vi "Xml_Fill_Default_Experiments.vi"(6 "error in (no error)":errorcluster, 9 "Resources Path":path=path "D:/PIRENEA/TECHNICAL/RESOURCES") -> (0 "error out":errorcluster caption="sortie d'erreur", 3 "EXPERIMENT Inputs":T1={"Setup"="", "Date"="", "User Name"="", "Comment"="", "Experiment Procedures"=[], "Chemical Source"="", "Sample Components"=[], "Species"=[], "Laser 1"={"Used"=TRUE, "Name"="Spectroscopy", "Wavelength"=1000.0, "Energy"=25.0}, "Laser 2"={"Used"=TRUE, "Name"="Spectroscopy", "Wavelength"=1000.0, "Energy"=25.0}, "Laser 3"={"Used"=TRUE, "Name"="Spectroscopy", "Wavelength"=1000.0, "Energy"=25.0}, "Laser 4"={"Used"=TRUE, "Name"="Spectroscopy", "Wavelength"=1000.0, "Energy"=25.0}, "Laser 5"={"Used"=TRUE, "Name"="Spectroscopy", "Wavelength"=1000.0, "Energy"=25.0}, "Lamp 1"={"Used"=TRUE, "Name"="Yag", "Wavelength"=1000.0, "Attenuation"=25.0}, "Lamp 2"={"Used"=TRUE, "Name"="Yag", "Wavelength"=1000.0, "Attenuation"=25.0}, "Gas 1"={"Used"=TRUE, "Name"="Yag", "Pressure"=1000.0}, "Gas 2"={"Used"=TRUE, "Name"="Yag", "Pressure"=1000.0}, "Gas 3"={"Used"=TRUE, "Name"="Yag", "Pressure"=1000.0}, "Gas 4"={"Used"=TRUE, "Name"="Spectroscopy", "Pressure"=1000.0}, "Gas 5"={"Used"=TRUE, "Name"="Spectroscopy", "Pressure"=1000.0}})   [LabVIEW 2018]
doc: "This example demonstrates how to convert a LabVIEW data structure into an XML string using the GXML reference library."
uses:
  controls/EXPERIMENT_Inputs.ctl
  controls/LASER_Inputs.ctl
  controls/LAMP_Inputs.ctl
  controls/GAS_Inputs.ctl
  <vilib>/Utility/config.llb/Read Key (String).vi
  <vilib>/Utility/config.llb/NI_LVConfig.lvlib
panel:
  in  "Chemical Source":string(combo)
  in  "Setup":string
  in  "Species":i32[](listbox)
  in  "Sample Components":i32[](listbox)
  in  "Procedures":i32[](listbox)
  in  "Users":string(combo)
  # "Lasers"
  # "nm"
  # "mJ"
  # "Lamps"
  # "nm"
  # "dB"
  # "Gas"
  # "bar"
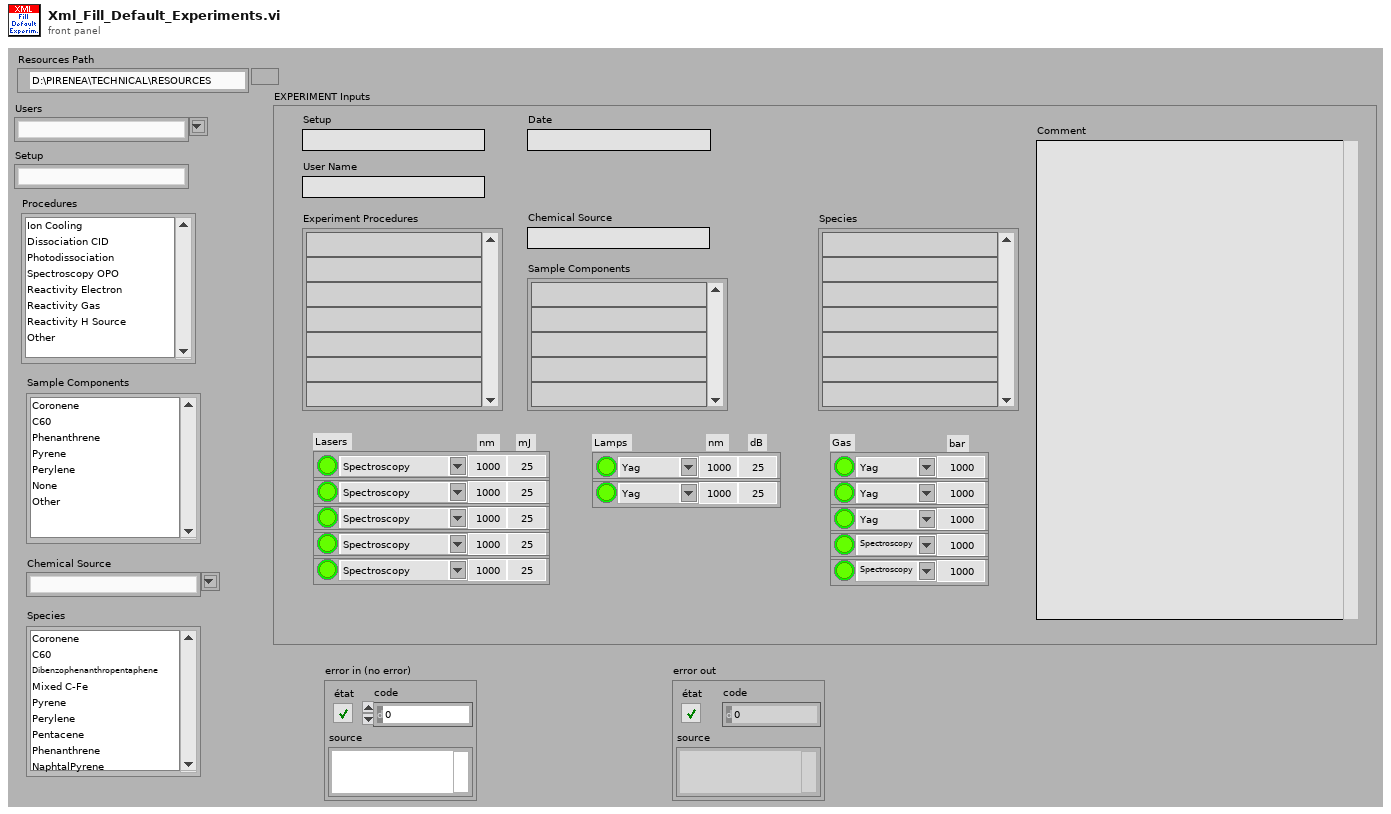
[diagram p1: front panel]
types:
  T1 = typedef "EXPERIMENT_Inputs.ctl" = cluster{"Setup":string, "Date":string, "User Name":string, "Comment":string, "Experiment Procedures":string[], "Chemical Source":string, "Sample Components":string[], "Species":string[], "Laser 1":T2, "Laser 2":T2, "Laser 3":T2, "Laser 4":T2, "Laser 5":T2, "Lamp 1":T3, "Lamp 2":T3, "Gas 1":T4, "Gas 2":T4, "Gas 3":T4, "Gas 4":T4, "Gas 5":T4}
  T2 = typedef "LASER_Inputs.ctl" = cluster{"Used":bool, "Name":string, "Wavelength":dbl, "Energy":dbl}
  T3 = typedef "LAMP_Inputs.ctl" = cluster{"Used":bool, "Name":string, "Wavelength":dbl, "Attenuation":dbl}
  T4 = typedef "GAS_Inputs.ctl" = cluster{"Used":bool, "Name":string, "Pressure":dbl}
  T5 = typedef "NI_LVConfig.lvlib/Config Data RefNum.ctl" = refnum<k1>
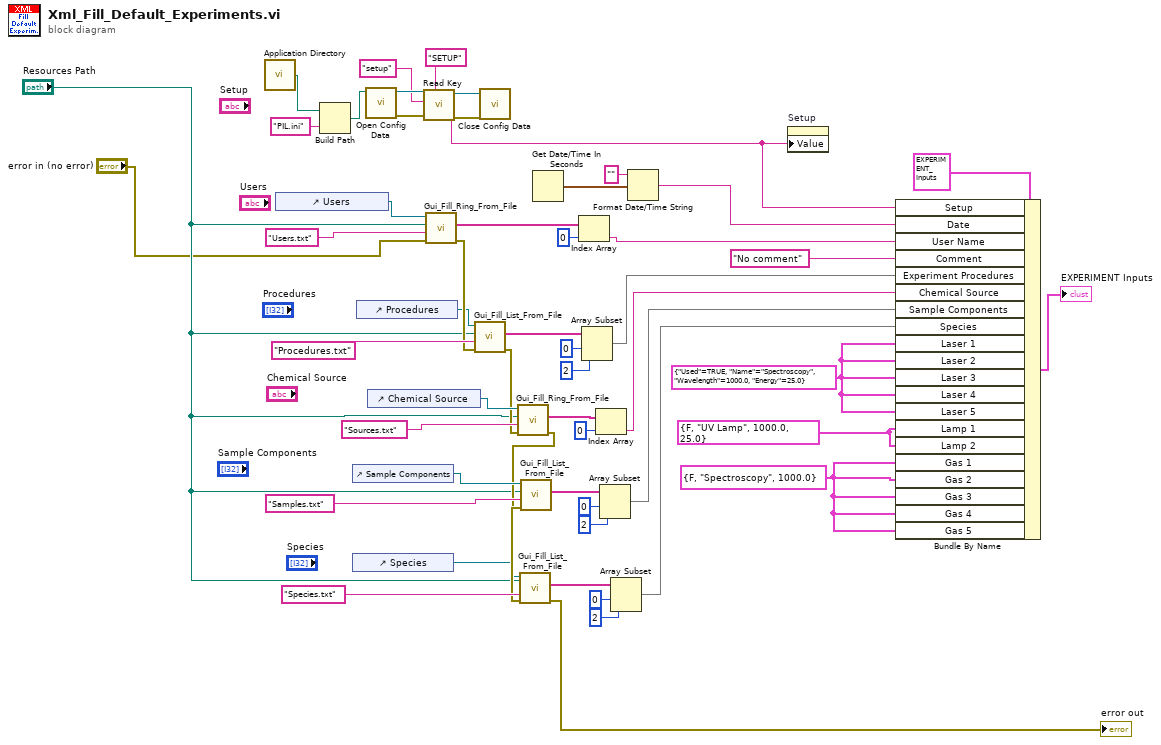
[diagram p0: block diagram]
diagram:
  w12 = T4 {"Used"=FALSE, "Name"="Spectroscopy", "Pressure"=1000.0} ("Gas 1")
  w13 = T3 {"Used"=FALSE, "Name"="UV Lamp", "Wavelength"=1000.0, "Attenuation"=25.0} ("Lamp 1")
  w25 = T2 {"Used"=TRUE, "Name"="Spectroscopy", "Wavelength"=1000.0, "Energy"=25.0} ("Laser 1")
  n1 = call <vilib>:"Application Directory.vi"() -> ("Application Directory"=w10:path)
  n2 = control-ref of="Users"() -> (w29:refnum<vi>)
  n3 = Build Path(base path=w10, name or relative path="PIL.ini" ("nom ou chemin relatif")) -> (appended path=w8:path)
  n4 = control-ref of="Sample Components"() -> (w27:refnum<vi>)
  n5 = control-ref of="Species"() -> (w26:refnum<vi>)
  n6 = control-ref of="Procedures"() -> (w28:refnum<vi>)
  n7 = call <vilib>:"Open Config Data.vi"("configuration file path"=w8) -> ("error out"=w2:errorcluster, "refnum"=w7:T5)  [unwired: 8 in, 1 out]
  n8 = control-ref of="Chemical Source"() -> (w21:refnum<vi>)
  n9 = call-poly <vilib>:"Read Key.vi"("section"="SETUP", "error in (no error)"=w2, "key"="setup", "refnum"=w7) -> ("error out"=w3:errorcluster, "value"=w1:string, "refnum out"=w4:T5)  [unwired: 4 in, 1 out]
  n10 = call "Gui_Fill_Ring_From_File.vi"("error in (no error)"="error in (no error)", "Resource Name"="Users.txt", "Resource Path"="Resources Path", "Refnum ChneDér"=w29) -> ("error out"=w46:errorcluster, "Table"=w52:string[])  [unwired: 4 in, 2 out]
  n11 = call "Gui_Fill_List_From_File.vi"("error in (no error)"=w46, "Resource Name"="Procedures.txt", "Resource Path"="Resources Path", "Refnum LstDér"=w28) -> ("error out"=w20:errorcluster, "Table"=w45:string[])  [unwired: 5 in, 1 out]
  n12 = call <vilib>:"Close Config Data.vi"("error in (no error)"=w3, "refnum"=w4) -> ()  [unwired: 8 in, 2 out]
  n13 = call "Gui_Fill_Ring_From_File.vi"("error in (no error)"=w20, "Resource Name"="Sources.txt", "Resource Path"="Resources Path", "Refnum ChneDér"=w21) -> ("error out"=w16:errorcluster, "Table"=w18:string[])  [unwired: 4 in, 2 out]
  n14 = call "Gui_Fill_List_From_File.vi"("error in (no error)"=w16, "Resource Name"="Samples.txt", "Resource Path"="Resources Path", "Refnum LstDér"=w27) -> ("error out"=w31:errorcluster, "Table"=w39:string[])  [unwired: 5 in, 1 out]
  n15 = call "Gui_Fill_List_From_File.vi"("error in (no error)"=w31, "Resource Name"="Species.txt", "Resource Path"="Resources Path", "Refnum LstDér"=w26) -> ("error out"=→"error out":errorcluster, "Table"=w35:string[])  [unwired: 5 in, 1 out]
  n16 = Get Date/Time In Seconds() -> (seconds since 1Jan1904=w50:timestamp)
  n17 = Index Array(array=w52, index=0 ("indice")) -> (element=w23:string)
  n18 = Array Subset(array=w45, index=0 ("indice"), length=2 ("longueur")) -> (w42:string[])
  n19 = Index Array(array=w18, index=0 ("indice")) -> (element=w17:string)
  n20 = Array Subset(array=w39, index=0 ("indice"), length=2 ("longueur")) -> (w37:string[])
  n21 = Array Subset(array=w35, index=0 ("indice"), length=2 ("longueur")) -> (w32:string[])
  n22 = Format Date/Time String(time format string (%c)="" ("chaîne de format de l'heure (%c)"), seconds (now)=w50) -> (date/time string=w24:string)  [unwired: 1 in]
  n23 = property on="Setup" class="Ch"("Value"=w1) -> ()  [unwired: 2 in, 2 out]
  n24 = Bundle By Name(cluster=T1 {"Setup"="", "Date"="", "User Name"="", "Comment"="", "Experiment Procedures"=[], "Chemical Source"="", "Sample Components"=[], "Species"=[], "Laser 1"={"Used"=TRUE, "Name"="Spectroscopy", "Wavelength"=1000.0, "Energy"=25.0}, "Laser 2"={"Used"=TRUE, "Name"="Spectroscopy", "Wavelength"=1000.0, "Energy"=25.0}, "Laser 3"={"Used"=TRUE, "Name"="Spectroscopy", "Wavelength"=1000.0, "Energy"=25.0}, "Laser 4"={"Used"=TRUE, "Name"="Spectroscopy", "Wavelength"=1000.0, "Energy"=25.0}, "Laser 5"={"Used"=TRUE, "Name"="Spectroscopy", "Wavelength"=1000.0, "Energy"=25.0}, "Lamp 1"={"Used"=TRUE, "Name"="Yag", "Wavelength"=1000.0, "Attenuation"=25.0}, "Lamp 2"={"Used"=TRUE, "Name"="Yag", "Wavelength"=1000.0, "Attenuation"=25.0}, "Gas 1"={"Used"=TRUE, "Name"="Yag", "Pressure"=1000.0}, "Gas 2"={"Used"=TRUE, "Name"="Yag", "Pressure"=1000.0}, "Gas 3"={"Used"=TRUE, "Name"="Yag", "Pressure"=1000.0}, "Gas 4"={"Used"=TRUE, "Name"="Spectroscopy", "Pressure"=1000.0}, "Gas 5"={"Used"=TRUE, "Name"="Spectroscopy", "Pressure"=1000.0}} ("EXPERIMENT Inputs"), "Setup"=w1, "Date"=w24, "User Name"=w23, "Comment"="No comment", "Experiment Procedures"=w42, "Chemical Source"=w17, "Sample Components"=w37, "Species"=w32, "Laser 1"=w25, "Laser 2"=w25, "Laser 3"=w25, "Laser 4"=w25, "Laser 5"=w25, "Lamp 1"=w13, "Lamp 2"=w13, "Gas 1"=w12, "Gas 2"=w12, "Gas 3"=w12, "Gas 4"=w12, "Gas 5"=w12) -> (→"EXPERIMENT Inputs":T1)
